vi "ET2604 - Write Temperature.vi"(0 "VISA resource name":refnum<visa-resource-name>, 7 "Data (0)":sgl format="%.3f", 11 "error in (no error)":errorcluster) -> (4 "VISA resource name out":refnum<visa-resource-name>, 15 "error out":errorcluster)   [LabVIEW 2017]
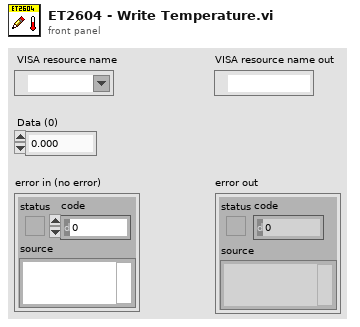
[diagram p1: front panel]
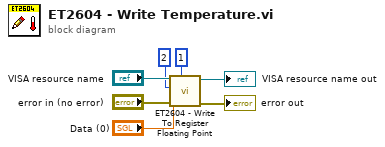
[diagram p0: block diagram]
diagram:
  n1 = call "ET2604 - Write To Register Floating Point.vi"("Unit Address (1)"=u8 1, "error in (no error)"="error in (no error)", "Data (0)"="Data (0)", "Register Address (0)"=u16 2, "VISA session"="VISA resource name") -> ("error out"=→"error out":errorcluster, "dup VISA session"=→"VISA resource name out":refnum<visa-resource-name>)  [unwired: 5 in]
